vi "Global 1.vi"() -> ()   [LabVIEW 2014]
panel:
  out "Date and Time to Print":string
  out "Date and Time":string
  out "Operator":string
  out "Serial Number 2":string
  out "Serial Number 1":string
  out "Data Buffer 2":string[](array[string])
  out "Data Buffer 1":string[](array[string])
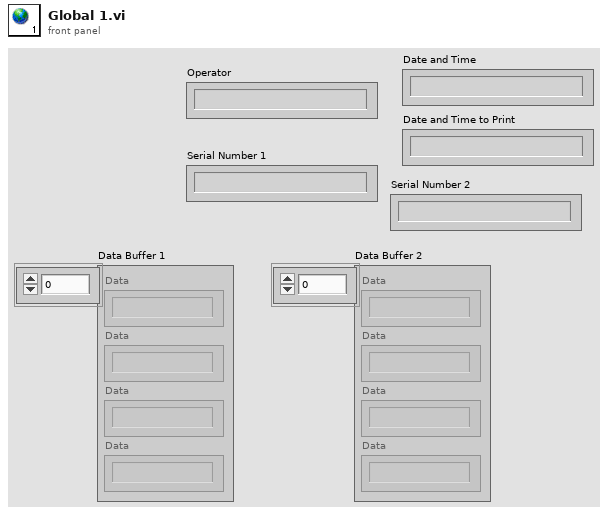
[diagram p1: front panel]
diagram:
